vi "U32toU64.vi"(6 "ready for output":bool, 9 "input valid":bool, 11 "U32 in":u32) -> (1 "output valid":bool, 3 "U64 out":u64, 4 "ready for input":bool)   [LabVIEW 2016]
doc: "Packing two U32 data into one U64"
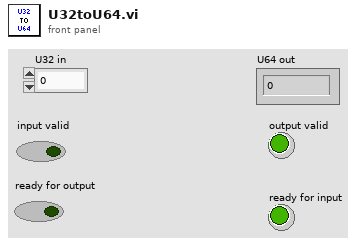
[diagram p1: front panel]
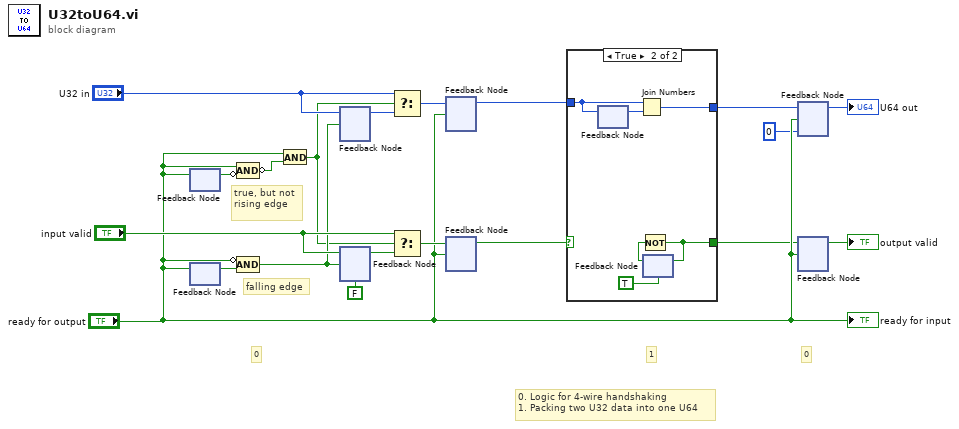
[diagram p0: block diagram]
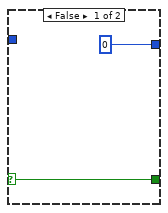
[diagram p2: hidden frame]
diagram:
  # "0. Logic for 4-wire handshaking\n1. Packing two U32 data into one U64"
  # "1"
  # "0"
  # "0"
  # "falling edge"
  # "true, but not rising edge"
  n1 = feedback-in #1("ready for output") -> ()
  n2 = feedback #1() -> (w17:bool)  [unwired: 1 in]
  n3 = feedback #2() -> (w16:bool)  [unwired: 1 in]
  n4 = feedback-in #2("ready for output") -> ()
  n5 = Compound Arithmetic op=AND("ready for output", invert w17) -> (invert w18:bool)
  n6 = Compound Arithmetic op=AND(invert "ready for output", w16) -> (w13:bool)
  n7 = And(x="ready for output", y=w18) -> (x .and. y?=w12:bool)
  n8 = feedback #3() -> (w19:u32)  [unwired: 1 in]
  n9 = feedback-in #3("U32 in", w13) -> ()
  n10 = feedback #4(FALSE) -> (w15:bool)
  n11 = feedback-in #4("input valid", w13) -> ()
  n12 = Select(t="U32 in", s=w12, f=w19) -> (s? t:f=w10:u32)
  n13 = Select(t="input valid", s=w12, f=w15) -> (s? t:f=w9:bool)
  n14 = feedback #5() -> (w5:u32)  [unwired: 1 in]
  n15 = feedback-in #5(w10, "ready for output") -> ()
  n16 = feedback #6() -> (w6:bool)  [unwired: 1 in]
  n17 = feedback-in #6(w9, "ready for output") -> ()
  n18 = case shown="True" w6 {
    selector: w6 -> [w22 _]
    tunnel: w5 -> [_ w28]
    tunnel: [w22 w24] -> w4
    tunnel: [u64 0 w23] -> w2
    frame False {
    }
    frame True {
      n19 = feedback #7() -> (w27:u32)  [unwired: 1 in]
      n20 = feedback-in #7(w28) -> ()
      n21 = Join Numbers(hi=w28, lo=w27) -> ((hi.lo)=w23:u64)
      n22 = feedback #8(TRUE) -> (w26:bool)
      n23 = Not(x=w26) -> (.not. x?=w24:bool)
      n24 = feedback-in #8(w24) -> ()
    }
  }
  n25 = feedback #9(u64 0 ("(hi.lo)")) -> (→"U64 out":u64)
  n26 = feedback-in #9(w2, "ready for output") -> ()
  n27 = feedback #10() -> (→"output valid":bool)  [unwired: 1 in]
  n28 = feedback-in #10(w4, "ready for output") -> ()
  "ready for input" <- "ready for output"
